vi "LVClass_ClosedLoopSmoothing_Ctor_FromMediumDefaultParams.vi"(0 "ClosedLoopSmoothing in":refnum<class "ClosedLoopSmoothing.lvclass">, 11 "error in (no error)":errorcluster) -> (4 "ClosedLoopSmoothing out":refnum<class "ClosedLoopSmoothing.lvclass">, 15 "error out":errorcluster)   [LabVIEW 2020, in "ClosedLoopSmoothing.lvclass"]
uses:
  ClosedLoopSmoothing.lvclass
  Handle creation.ctl
  ClosedLoopSmoothing.lvclass/ClosedLoopSmoothing.ctl
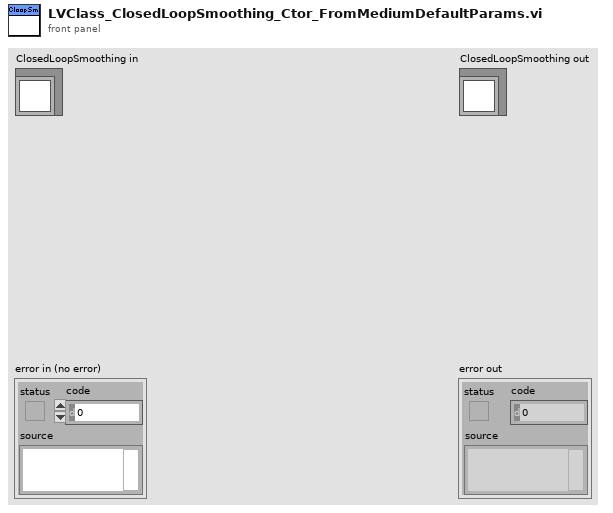
[diagram p1: front panel]
types:
  T1 = typedef "Handle creation.ctl" = enum16{"By ctor", "By write function"}
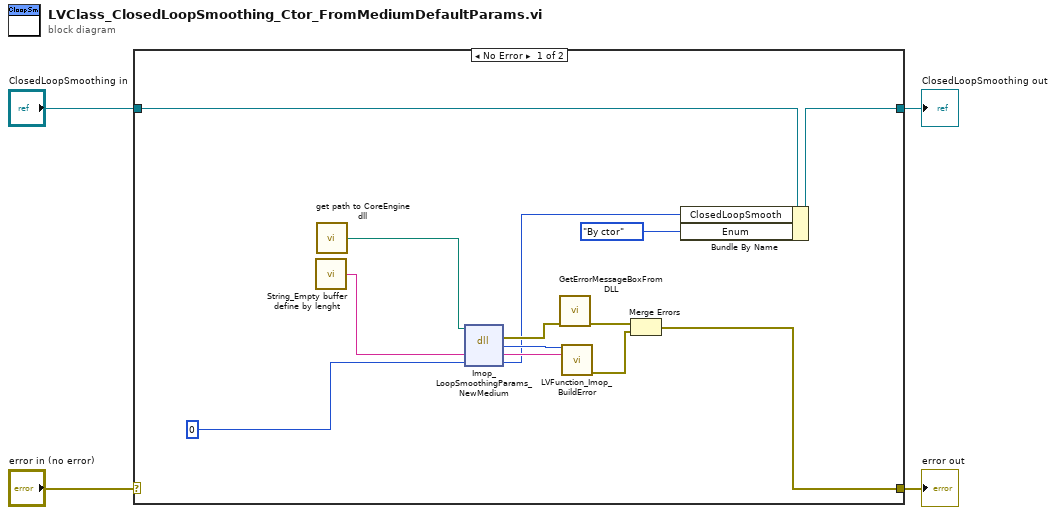
[diagram p0: block diagram]
diagram:
  n1 = case shown="No Error" "error in (no error)" {
    selector: "error in (no error)" -> [_ w19]
    tunnel: [w5 w19] -> w3
    tunnel: [w6 w18] -> w1
    tunnel: "ClosedLoopSmoothing in" -> [w7 w18]
    frame No Error {
      n2 = call "String_Empty buffer define by lenght.vi"() -> ("Empty buffer"=w17:string)  [unwired: 1 in]
      n3 = call "get path to CoreEngine dll.vi"() -> ("path to c_interface_vc100.dll"=w8:path)  [unwired: 12 in, 3 out]
      n4 = dll-call lib="D:/soft/HASO_v3/SVN_trunk/ImOpCoreEngine4_LV2011/DLLs/c_interface_vc100.dll" fn="Imop_LoopSmoothingParams_NewMedium"(path in=w8, "message"=w17, "smoothing_params"=0 ("Pupil")) -> (error out=w14:errorcluster, "return type"=w15:i32, "message"=w16:string, "smoothing_params"=w12:i32)  [unwired: 2 in, 1 out]
      n5 = call "GetErrorMessageBoxFromDLL.vi"("error IN"=w14) -> ("error OUT"=w10:errorcluster)  [unwired: 10 in]
      n6 = call "LVFunction_Imop_BuildError.vi"("code"=w15, "String to Prepend to source (\"\")"=w16) -> ("error out"=w9:errorcluster)  [unwired: 13 in]
      n7 = Merge Errors(w10, w9) -> (w5:errorcluster)
      n8 = Bundle By Name(cluster=w7, "ClosedLoopSmooth"=w12, "Enum"=Handle_creation."By ctor" ("Pupil ptr create")) -> (w6:refnum<class "ClosedLoopSmoothing.lvclass">)
    }
    frame Error {
    }
  }
  "error out" <- w3
  "ClosedLoopSmoothing out" <- w1
